vi "Update Position.vi"(8 "Direction":T1, 9 "Action":T2, 10 "Replicated in":refnum<class "64.lvclass">, 11 "64 in":refnum<class "64.lvclass">) -> (2 "Replicated out":refnum<class "64.lvclass">, 3 "64 out":refnum<class "64.lvclass">)   [LabVIEW 2015, in "64.lvclass"]
uses:
  64.lvclass
  Type Defs/Action Enum.ctl
  Type Defs/Direction Enum.ctl
  64.lvclass/64.ctl
  Square/Board Size.vi
  SubVIs/Read-Only Globals.vi
  SubVIs/Globals (private).vi
  Common/Common.lvlib
  Type Defs/SB Type Defs.lvlib
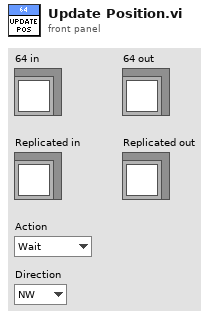
[diagram p1: front panel]
types:
  T1 = typedef "SB Type Defs.lvlib/Direction Enum.ctl" = enum16{"NW", "N", "NE", "E", "SE", "S", "SW", "W"}
  T2 = typedef "SB Type Defs.lvlib/Action Enum.ctl" = enum16{"Wait", "Move", "Attack", "Replicate"}
  T3 = typedef "Common.lvlib/Position.ctl" = cluster{"Column":i32, "Row":i32}
  T4 = typedef "Common.lvlib/Map DVR.ctl" = refnum<data-value>
  T5 = typedef "Common.lvlib/Location Data.ctl" = cluster{"Location State":enum16{"Empty", "Enemy", "Attacked", "Occupied"}}
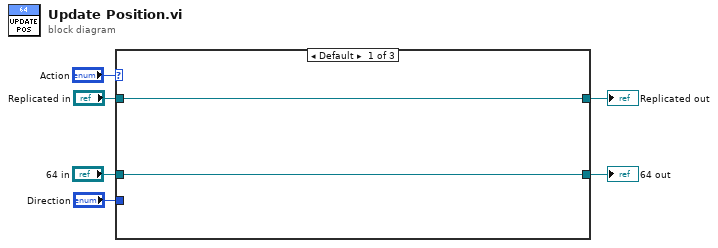
[diagram p0: block diagram]
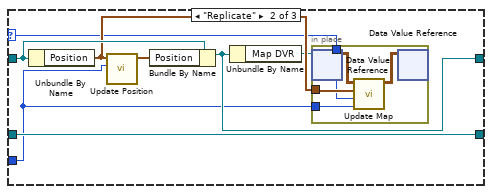
[diagram p2: hidden frame]
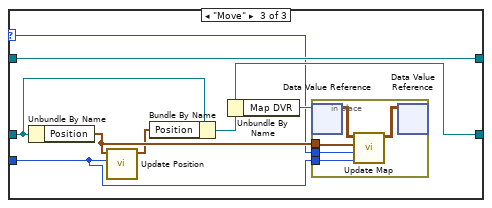
[diagram p3: hidden frame]
diagram:
  n1 = case shown="Default" "Action" {
    selector: "Action" -> [_ w9 w22]
    tunnel: "Replicated in" -> [w7 w16 w28]
    tunnel: "Direction" -> [_ w10 w23]
    tunnel: [w7 w12 w28] -> w3
    tunnel: "64 in" -> [w8 w15 w29]
    tunnel: [w8 w15 w25] -> w1
    frame Default {
    }
    frame "Replicate" {
      n2 = Unbundle By Name(w16) -> ("Position"=w14:T3)
      n3 = call "Update Position.vi"("Direction"=w10, "Position in"=w14) -> ("Position out"=w13:T3)  [unwired: 9 in]
      n4 = Bundle By Name(cluster=w16, "Position"=w13) -> (w12:refnum<class "64.lvclass">)
      n5 = Unbundle By Name(w12) -> ("Map DVR"=w11:T4)
      n6 = in-place {
        in-place-border: w14 -> [w21]
        in-place-border: w10 -> [w18]
        in-place-border: w9 -> [w17]
        n7 = in-place-dvr #1(w11) -> (w20:T5[][])  [unwired: 1 out]
        n8 = call "Update Map.vi"("Direction"=w18, "Action"=w17, "Old Position"=w21, "Map in"=w20) -> ("Map out"=w19:T5[][])  [unwired: 7 in]
        n9 = in-place-dvr #1(w19) -> ()  [unwired: 2 out]
      }
    }
    frame "Move" {
      n10 = Unbundle By Name(w29) -> ("Position"=w27:T3)
      n11 = call "Update Position.vi"("Direction"=w23, "Position in"=w27) -> ("Position out"=w26:T3)  [unwired: 9 in]
      n12 = Bundle By Name(cluster=w29, "Position"=w26) -> (w25:refnum<class "64.lvclass">)
      n13 = Unbundle By Name(w25) -> ("Map DVR"=w24:T4)
      n14 = in-place {
        in-place-border: w27 -> [w34]
        in-place-border: w23 -> [w31]
        in-place-border: w22 -> [w30]
        n15 = in-place-dvr #2(w24) -> (w33:T5[][])  [unwired: 1 out]
        n16 = call "Update Map.vi"("Direction"=w31, "Action"=w30, "Old Position"=w34, "Map in"=w33) -> ("Map out"=w32:T5[][])  [unwired: 7 in]
        n17 = in-place-dvr #2(w32) -> ()  [unwired: 2 out]
      }
    }
  }
  "64 out" <- w1
  "Replicated out" <- w3
